vi "Script Init VI.vi"(8 "error in":errorcluster, 9 "Ref.Init VI":refnum<vi>, 10 "Conpane Map":T1(c390)) -> (0 "error out":errorcluster)   [LabVIEW 2020, in "_Msg Rescript.lvlib" / "_Msg Rescript.lvclass"]
uses:
  _Msg Rescript.lvclass
  <vilib>/Utility/traverseref.llb/TRef TravTarget.ctl
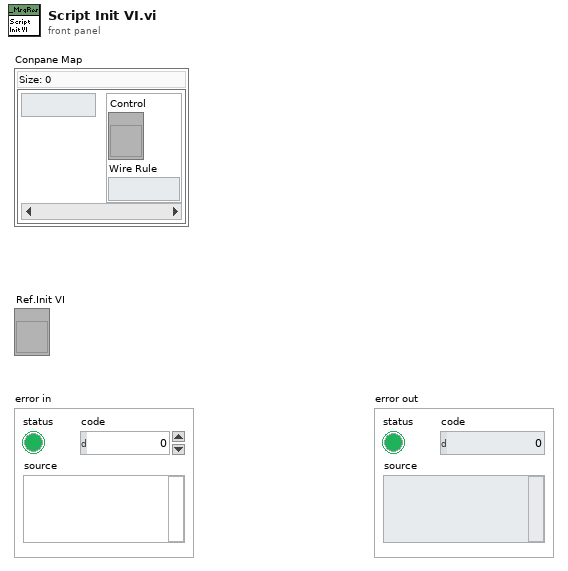
[diagram p1: front panel]
types:
  T1 = map{i32, cluster{"Control":refnum<vi>, "Wire Rule":enum16{"Invalid Wire Rule", "Required", "Recommended", "Optional", "Dynamic Dispatch"}}}
  T2 = typedef "TRef TravTarget.ctl" = enum16{"FP", "BD", "Other"}
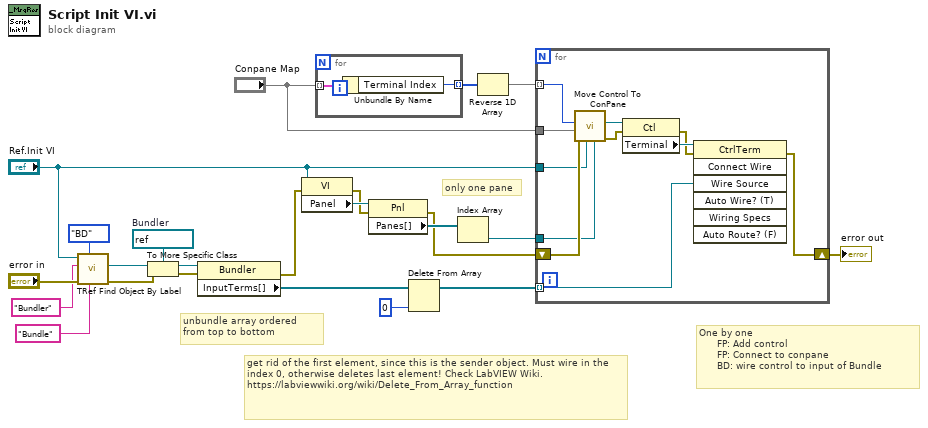
[diagram p0: block diagram]
diagram:
  w10 = refnum<vi> refnum  # Bundler
  # "get rid of the first element, since this is the sender object. Must wire in the index 0, otherwise deletes last element! Check LabVIEW Wiki.\nhttps://labviewwiki.org/wiki/Delete_From_Array_function"
  # "unbundle array ordered from top to bottom"
  # "One by one\n      FP: Add control\n      FP: Connect to conpane\n      BD: wire control to input of Bundle"
  # "only one pane"
  n1 = call <vilib>:"TRef Find Object By Label.vi"("Label"="Bundle", "Traverse Target"=TRef_TravTarget."BD", "error in (no error)"="error in", "Class Name"="Bundler", "VI Ref"="Ref.Init VI") -> ("error out"=w14:errorcluster, "Found Obj Ref"=w13:refnum<vi>)  [unwired: 3 in, 2 out]
  n2 = To More Specific Class(target class=w10, reference=w13, error in=w14) -> (specific class reference=w8:refnum<vi>, error out=w7:errorcluster)
  n3 = property class="Bundler"(reference=w8, error in=w7) -> (error out=w19:errorcluster, "InputTerms[]"=w5:refnum<vi>[])  [unwired: 1 out]
  n4 = property class="VI"(reference="Ref.Init VI", error in=w19) -> (error out=w18:errorcluster, "Panel"=w21:refnum<vi>)  [unwired: 1 out]
  n5 = for {
    tunnel: "Conpane Map" -> [w25] mode=indexing
    tunnel: [w24] -> w23 mode=indexing
    n6 = Unbundle By Name(w25) -> ("Terminal Index"=w24:i32)
  }
  n7 = property class="Pnl"(reference=w21, error in=w18) -> (error out=w17:errorcluster, "Panes[]"=w20:refnum<vi>[])  [unwired: 1 out]
  n8 = Delete From Array(array=w5, index=0) -> (array with subset deleted=w2:refnum<vi>[])  [unwired: 1 in, 1 out]
  n9 = Index Array(array=w20) -> (element=w16:refnum<vi>)  [unwired: 1 in]
  n10 = Reverse 1D Array(array=w23) -> (reversed array=w22:i32[])
  n11 = for {
    tunnel: w22 -> [w30] mode=indexing
    tunnel: "Conpane Map" -> [w27]
    tunnel: w16 -> [w28]
    tunnel: "Ref.Init VI" -> [w26]
    tunnel: w2 -> [w35] mode=indexing
    shift-right: [w33] -> w4
    shift-left: w17 -> [w29]
    n12 = call "Move Control To ConPane.vi"("Pane"=w28, "Ref. VI"=w26, "error in"=w29, "Conpane Map"=w27, "Terminal Index"=w30) -> ("error out"=w31:errorcluster, "Control"=w32:refnum<vi>)  [unwired: 5 in]
    n13 = property class="Ctl"(reference=w32, error in=w31) -> (error out=w34:errorcluster, "Terminal"=w36:refnum<vi>)  [unwired: 1 out]
    n14 = invoke class="CtrlTerm" method="Connect Wire"(reference=w36, error in=w34, "Wire Source"=w35) -> (error out=w33:errorcluster)  [unwired: 4 in, 6 out]
  }
  "error out" <- w4
